vi "ObjectHandler.AddReference.vi"(8 "error in (no error)":errorcluster, 10 "ObjectMessage":T1={"Name"="", "ObjectWType"={"ObjectType"=enum."ObjectHandler", "Object"=variant(refnum<data-value> refnum)}}, 11 "ObjectHandler in":refnum<class "ObjectHandler.lvclass">) -> (0 "error out":errorcluster, 3 "ObjectHandler out":refnum<class "ObjectHandler.lvclass">)   [LabVIEW 2016, in "ObjectHandler.lvclass"]
uses:
  ObjectHandler.lvclass
  ObjectHandler.ObjectMessage.ctl
  ObjectHandler.ObjectWType.ctl
  ObjectHandler.ObjectType.ctl
  ViHandler/ViHandler.lvclass
  Package ErrorHandling/ErrorHandling.lvclass
  CentralStorage/CentralStorage.lvclass
  Package Simulation/Modell/Hausmodell/Hausmodell.lvclass
  Package Simulation/Modell/Sondenmodell/Sondenmodell.lvclass
  Package Simulation/Modell/Umgebung/Umgebung.lvclass
  ObjectHandler.lvclass/ObjectHandler.ctl
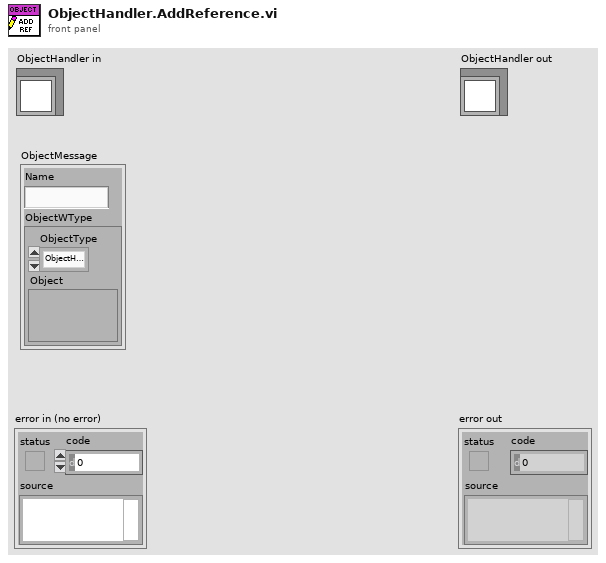
[diagram p1: front panel]
types:
  T1 = typedef "ObjectHandler.lvclass/ObjectHandler.ObjectMessage.ctl" = cluster{"Name":string, "ObjectWType":T2}
  T2 = typedef "ObjectHandler.lvclass/ObjectHandler.ObjectWType.ctl" = cluster{"ObjectType":T3, "Object":variant}
  T3 = typedef "ObjectHandler.lvclass/ObjectHandler.ObjectType.ctl" = enum16{"undefined", "ObjectHandler", "ViHandler", "ErrorHandler", "CentralStorage", "Hausmodell", "Sondenmodell", "Wärmepumpe", "Umgebung"}
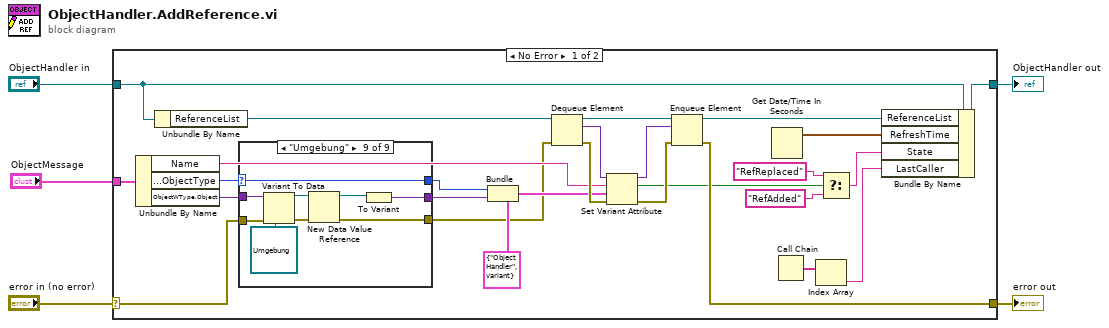
[diagram p0: block diagram]
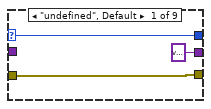
[diagram p2: hidden frame]
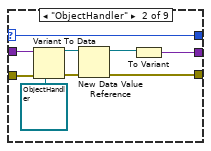
[diagram p3: hidden frame]
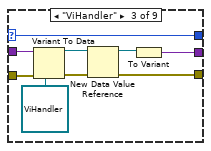
[diagram p4: hidden frame]
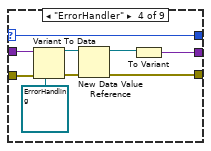
[diagram p5: hidden frame]
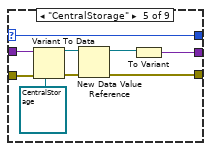
[diagram p6: hidden frame]
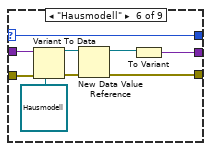
[diagram p7: hidden frame]
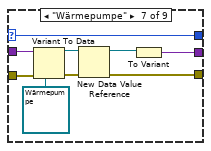
[diagram p8: hidden frame]
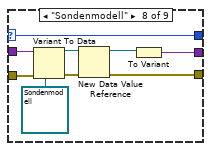
[diagram p9: hidden frame]
diagram:
  n1 = case shown="No Error" "error in (no error)" {
    selector: "error in (no error)" -> [w8 w108]
    tunnel: [w23 w108] -> w4
    tunnel: [w32 w109] -> w2
    tunnel: "ObjectHandler in" -> [w31 w109]
    tunnel: "ObjectMessage" -> [w28 _]
    frame No Error {
      n2 = Unbundle By Name(w28) -> ("Name"=w18:string, "ObjectWType.ObjectType"=w11:T3, "ObjectWType.Object"=w9:variant)
      n3 = Unbundle By Name(w31) -> ("ReferenceList"=w25:refnum<queue>)
      n4 = case shown="\"Umgebung\"" w11 {
        selector: w11 -> [w35 w44 w53 w62 w71 w80 w89 w98 w107]
        tunnel: [w35 w44 w53 w62 w71 w80 w89 w98 w107] -> w10
        tunnel: w9 -> [_ w43 w52 w61 w70 w79 w88 w97 w106]
        tunnel: w8 -> [w33 w38 w48 w57 w67 w76 w85 w94 w103]
        tunnel: [w33 w37 w47 w56 w66 w75 w84 w93 w102] -> w7
        tunnel: [variant ("Variant") w36 w46 w55 w65 w74 w83 w92 w101] -> w6
        frame "undefined", Default {
        }
        frame "ObjectHandler" {
          n5 = Variant To Data(error in=w38, type=refnum<class "ObjectHandler.lvclass"> refnum ("ObjectHandler.lvclass"), Variant=w43) -> (data=w41:refnum<class "ObjectHandler.lvclass">, error out=w39:errorcluster)
          n6 = New Data Value Reference(data value=w41, error in=w39) -> (data value reference=w40:refnum<data-value>, error out=w37:errorcluster)
          n7 = To Variant(anything=w40) -> (Variant=w36:variant)
        }
        frame "ViHandler" {
          n8 = Variant To Data(error in=w48, type=refnum<class "ViHandler.lvclass"> refnum ("ViHandler.lvclass"), Variant=w52) -> (data=w51:refnum<class "ViHandler.lvclass">, error out=w49:errorcluster)
          n9 = New Data Value Reference(data value=w51, error in=w49) -> (data value reference=w50:refnum<data-value>, error out=w47:errorcluster)
          n10 = To Variant(anything=w50) -> (Variant=w46:variant)
        }
        frame "ErrorHandler" {
          n11 = Variant To Data(error in=w57, type=refnum<class "ErrorHandling.lvclass"> refnum ("ErrorHandling.lvclass"), Variant=w61) -> (data=w60:refnum<class "ErrorHandling.lvclass">, error out=w58:errorcluster)
          n12 = New Data Value Reference(data value=w60, error in=w58) -> (data value reference=w59:refnum<data-value>, error out=w56:errorcluster)
          n13 = To Variant(anything=w59) -> (Variant=w55:variant)
        }
        frame "CentralStorage" {
          n14 = Variant To Data(error in=w67, type=refnum<class "CentralStorage.lvclass"> refnum ("CentralStorage.lvclass"), Variant=w70) -> (data=w64:refnum<class "CentralStorage.lvclass">, error out=w68:errorcluster)
          n15 = New Data Value Reference(data value=w64, error in=w68) -> (data value reference=w69:refnum<data-value>, error out=w66:errorcluster)
          n16 = To Variant(anything=w69) -> (Variant=w65:variant)
        }
        frame "Hausmodell" {
          n17 = Variant To Data(error in=w76, type=refnum<class "Hausmodell.lvclass"> refnum ("Hausmodell.lvclass"), Variant=w79) -> (data=w73:refnum<class "Hausmodell.lvclass">, error out=w77:errorcluster)
          n18 = New Data Value Reference(data value=w73, error in=w77) -> (data value reference=w78:refnum<data-value>, error out=w75:errorcluster)
          n19 = To Variant(anything=w78) -> (Variant=w74:variant)
        }
        frame "Wärmepumpe" {
          n20 = Variant To Data(error in=w85, type=refnum<class "Wärmepumpe.lvclass"> refnum ("Wärmepumpe.lvclass"), Variant=w88) -> (data=w82:refnum<class "Wärmepumpe.lvclass">, error out=w86:errorcluster)
          n21 = New Data Value Reference(data value=w82, error in=w86) -> (data value reference=w87:refnum<data-value>, error out=w84:errorcluster)
          n22 = To Variant(anything=w87) -> (Variant=w83:variant)
        }
        frame "Sondenmodell" {
          n23 = Variant To Data(error in=w94, type=refnum<class "Sondenmodell.lvclass"> refnum ("Sondenmodell.lvclass"), Variant=w97) -> (data=w91:refnum<class "Sondenmodell.lvclass">, error out=w95:errorcluster)
          n24 = New Data Value Reference(data value=w91, error in=w95) -> (data value reference=w96:refnum<data-value>, error out=w93:errorcluster)
          n25 = To Variant(anything=w96) -> (Variant=w92:variant)
        }
        frame "Umgebung" {
          n26 = Variant To Data(error in=w103, type=refnum<class "Umgebung.lvclass"> refnum ("Umgebung.lvclass"), Variant=w106) -> (data=w100:refnum<class "Umgebung.lvclass">, error out=w104:errorcluster)
          n27 = New Data Value Reference(data value=w100, error in=w104) -> (data value reference=w105:refnum<data-value>, error out=w102:errorcluster)
          n28 = To Variant(anything=w105) -> (Variant=w101:variant)
        }
      }
      n29 = Bundle(cluster=T2 {"ObjectType"=enum."ObjectHandler", "Object"=variant} ("ObjectWType"), "ObjectType"=w10, "Object"=w6) -> (w17:T2)
      n30 = Dequeue Element(queue=w25, error in (no error)=w7) -> (queue out=w24:refnum<queue>, element=w22:variant, error out=w20:errorcluster)  [unwired: 1 in, 1 out]
      n31 = Set Variant Attribute(Variant=w22, name=w18, value=w17, error in=w20) -> (Variant out=w21:variant, replaced=w15:bool, error out=w19:errorcluster)
      n32 = Enqueue Element(queue=w24, element=w21, error in (no error)=w19) -> (queue out=w16:refnum<queue>, error out=w23:errorcluster)  [unwired: 1 in, 1 out]
      n33 = Get Date/Time In Seconds() -> (seconds since 1Jan1904=w29:timestamp)
      n34 = Call Chain() -> (call chain=w30:string[])
      n35 = Index Array(array=w30) -> (element=w27:string)  [unwired: 1 in]
      n36 = Select(t="RefReplaced" ("State"), s=w15, f="RefAdded" ("State")) -> (s? t:f=w12:string)
      n37 = Bundle By Name(cluster=w31, "ReferenceList"=w16, "RefreshTime"=w29, "State"=w12, "LastCaller"=w27) -> (w32:refnum<class "ObjectHandler.lvclass">)
    }
    frame Error {
    }
  }
  "error out" <- w4
  "ObjectHandler out" <- w2
